vi "Activate Version.vi"(6 "wait for reply (T)":bool=TRUE, 7 "ITSDiscovery.lvclass":refnum<class "ITSDiscovery.lvclass">, 8 "error in":errorcluster, 9 "IProcess Executor.lvclass":refnum<class "IProcess Executor.lvclass">, 10 "Version":string) -> (0 "error out":errorcluster, 1 "timed out?":bool)   [LabVIEW 2025, in "TS Environment Manager.lvlib"]
doc: "Activates the specified TS version.\n\n_____\nCreated using DQMH Framework: Event Scripter 7.1.1.1528."
uses:
  TS Environment Manager.lvlib
  IProcess Executor/IProcess Executor.lvclass
  ITSDiscovery/ITSDiscovery.lvclass
  Activate Version Argument--cluster.ctl
  Activate Version (Reply Payload)--cluster.ctl
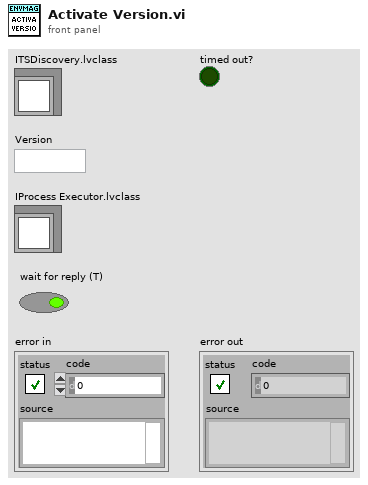
[diagram p1: front panel]
types:
  T1 = typedef "TS Environment Manager.lvlib/Activate Version Argument--cluster.ctl" = cluster{"Version":string, "IProcess Executor.lvclass":refnum<class "IProcess Executor.lvclass">, "ITSDiscovery.lvclass":refnum<class "ITSDiscovery.lvclass">, "Wait Notifier":refnum<notifier>, "wait for reply":bool}
  T2 = typedef "TS Environment Manager.lvlib/Request Events--cluster.ctl" = cluster{"Stop Module":refnum<user-event>, "Show Panel":refnum<user-event>, "Hide Panel":refnum<user-event>, "Get Module Execution Status":refnum<user-event>, "Show Diagram":refnum<user-event>, "Get Installations":refnum<user-event>, "Private.Get Profiles File":refnum<user-event>, "Launch Sequence Editor":refnum<user-event>, "Activate Version":refnum<user-event>, "Add Profile":refnum<user-event>, "Get Profile(s)":refnum<user-event>, "Delete Profile":refnum<user-event>, "Set Profiles File":refnum<user-event>}
  T3 = typedef "TS Environment Manager.lvlib/Activate Version (Reply Payload)--cluster.ctl" = cluster{"error":errorcluster, "Version":string}
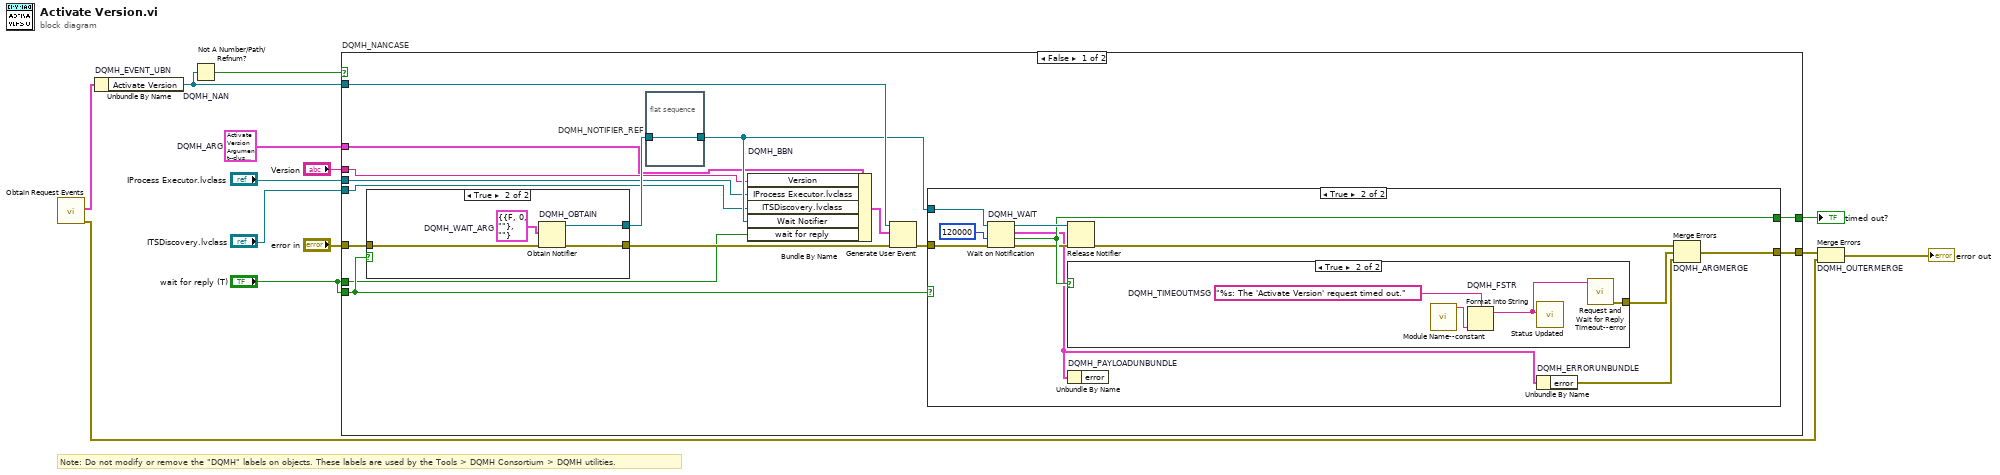
[diagram p0: block diagram]
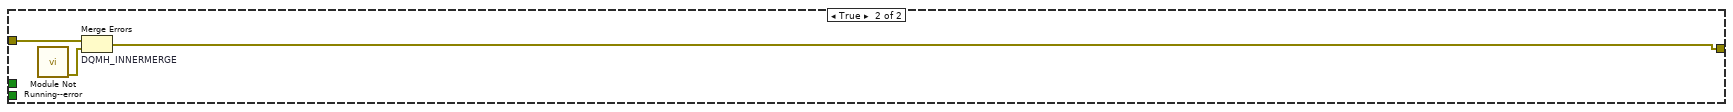
[diagram p5: hidden frame]
diagram:
  w7 = T1 {"Version"="", "IProcess Executor.lvclass"=refnum, "ITSDiscovery.lvclass"=refnum, "Wait Notifier"=refnum, "wait for reply"=FALSE}  # DQMH_ARG
  # "Note: Do not modify or remove the \"DQMH\" labels on objects. These labels are used by the Tools > DQMH Consortium > DQMH utilities."
  n1 = call "Obtain Request Events.vi"() -> ("error out"=w2:errorcluster, "TS Environment Manager Request Events"=w1:T2)  [unwired: 10 in]
  n2 = Unbundle By Name "DQMH_EVENT_UBN"(w1) -> ("Activate Version"=w8:refnum<user-event>)
  n3 = Not A Number/Path/Refnum? "DQMH_NAN"(number/path/refnum=w8) -> (NaN/Path/Refnum?=w9:bool)
  n4 = case "DQMH_NANCASE" shown="False" w9 {
    tunnel: "error in" -> [w28 w53]
    tunnel: w8 -> [w26 _]
    tunnel: [w23 w52] -> w10
    tunnel: [w24 _] -> w12
    tunnel: "wait for reply (T)" -> [w21 _]
    tunnel: w7 -> [w18 _]
    tunnel: "Version" -> [w17 _]
    tunnel: "IProcess Executor.lvclass" -> [w16 _]
    tunnel: "ITSDiscovery.lvclass" -> [w15 _]
    tunnel: "wait for reply (T)" -> [w14 _]
    frame False {
      n5 = case shown="True" w21 {
        tunnel: w28 -> [w46 w50]
        tunnel: [w46 w49] -> w25
        tunnel: [_ w47] -> w20
        frame False {
        }
        frame True {
          w48 = T3 {"error"={"status"=FALSE, "code"=0, "source"=""}, "Version"=""}  # DQMH_WAIT_ARG
          n6 = Obtain Notifier "DQMH_OBTAIN"(notification data type=w48, error in (no error)=w50) -> (notifier out=w47:refnum<notifier>, error out=w49:errorcluster)  [unwired: 2 in, 1 out]
        }
      }
      n7 = flat-sequence "DQMH_NOTIFIER_REF" {
        tunnel: w20 -> [w29]
        tunnel: [w29] -> w19
        frame #0 {
        }
      }
      n8 = Bundle By Name "DQMH_BBN"(cluster=w18, "Version"=w17, "IProcess Executor.lvclass"=w16, "ITSDiscovery.lvclass"=w15, "Wait Notifier"=w19, "wait for reply"=w14) -> (w22:T1)
      n9 = Generate User Event(user event=w26, event data cluster=w22, error in=w25) -> (error out=w27:errorcluster)  [unwired: 1 in, 1 out]
      n10 = case shown="True" w21 {
        tunnel: w27 -> [w30 w41]
        tunnel: w19 -> [_ w40]
        tunnel: [_ w38] -> w24
        tunnel: [w30 w37] -> w23
        frame False {
        }
        frame True {
          n11 = Wait on Notification "DQMH_WAIT"(notifier=w40, timeout in ms (-1)=120000, error in (no error)=w41) -> (notifier out=w39:refnum<notifier>, notification=w32:T3, timed out?=w38:bool, error out=w36:errorcluster)  [unwired: 1 in]
          n12 = Release Notifier(notifier=w39, error in (no error)=w36) -> (error out=w35:errorcluster)  [unwired: 1 in, 2 out]
          n13 = case shown="True" w38 {
            tunnel: [_ w43] -> w33
            frame False {
            }
            frame True {
              w45 = "%s: The 'Activate Version' request timed out."  # DQMH_TIMEOUTMSG
              n14 = call "Module Name--constant.vi"() -> ("Module Name"=w42:string)  [unwired: 11 in]
              n15 = Format Into String "DQMH_FSTR"(format string=w45, w42) -> (resulting string=w44:string)  [unwired: 2 in, 1 out]
              n16 = call "Status Updated.vi"("Status"=w44) -> ()  [unwired: 10 in, 1 out]
              n17 = call "Request and Wait for Reply Timeout--error.vi"("Error Message"=w44) -> ("error out"=w43:errorcluster)  [unwired: 10 in]
            }
          }
          n18 = Unbundle By Name "DQMH_PAYLOADUNBUNDLE"(w32) -> ()  [unwired: 1 out]
          n19 = Unbundle By Name "DQMH_ERRORUNBUNDLE"(w32) -> ("error"=w34:errorcluster)
          n20 = Merge Errors "DQMH_ARGMERGE"(w35, w33, w34) -> (w37:errorcluster)
        }
      }
    }
    frame True {
      n21 = call "Module Not Running--error.vi"() -> ("error out"=w51:errorcluster)  [unwired: 11 in]
      n22 = Merge Errors "DQMH_INNERMERGE"(w53, w51) -> (w52:errorcluster)
    }
  }
  "timed out?" <- w12
  n23 = Merge Errors "DQMH_OUTERMERGE"(w10, w2) -> (→"error out":errorcluster)
